vi "Lab1_Exercise3_SUBVI.vi"(9 "Numeric in":dbl, 10 "Number 1":dbl, 11 "Enum":T1(ring)) -> (2 "Error LED":bool, 3 "Numeric out":dbl)   [LabVIEW 2016]
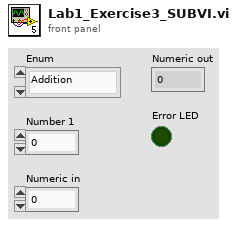
[diagram p1: front panel]
types:
  T1 = enum16{"Addition", "Subtraction", "Multiplication", "Division"}
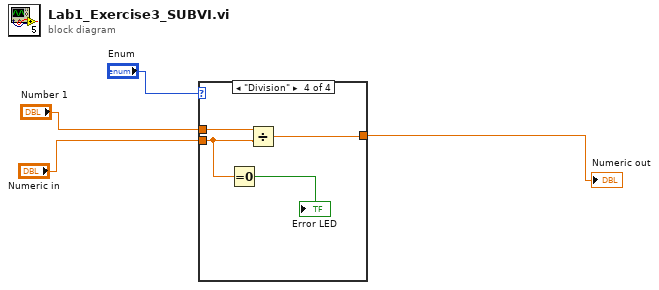
[diagram p0: block diagram]
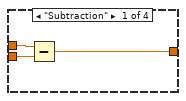
[diagram p2: hidden frame]
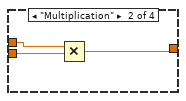
[diagram p3: hidden frame]
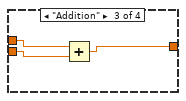
[diagram p4: hidden frame]
diagram:
  n1 = case shown="\"Division\"" "Enum" {
    tunnel: "Number 1" -> [w7 w10 w13 w17]
    tunnel: "Numeric in" -> [w6 w9 w12 w15]
    tunnel: [w5 w8 w11 w16] -> w3
    frame "Subtraction" {
      n2 = Subtract(x=w7, y=w6) -> (x-y=w5:dbl)
    }
    frame "Multiplication" {
      n3 = Multiply(x=w10, y=w9) -> (x*y=w8:dbl)
    }
    frame "Addition" {
      n4 = Add(x=w13, y=w12) -> (x+y=w11:dbl)
    }
    frame "Division" {
      n5 = Equal To 0?(x=w15) -> (x = 0?=→"Error LED":bool)
      n6 = Divide(x=w17, y=w15) -> (x/y=w16:dbl)
    }
  }
  "Numeric out" <- w3
